vi "Add NI-XNET CAN Hardware_Create Disable Signal.vi"(7 "SysDef Ref":T1, 8 "error in (no error)":errorcluster, 10 "Disable Node Path":string, 11 "Signal Based Frame":refnum<k24>) -> (0 "error out":errorcluster, 3 "Signal Based Frame out":refnum<k24>)   [LabVIEW 2019, in "Simple SysDef API.lvlib"]
uses:
  <userlib>/SimpleSysDef/Simple SysDef API.lvlib
  <userlib>/SimpleSysDef/_SubVIs/System Definition Reference.ctl
  NationalInstruments.VeriStand.SystemDefinitionAPI
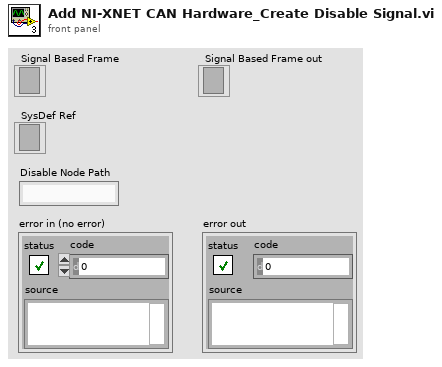
[diagram p1: front panel]
types:
  T1 = typedef "Simple SysDef API.lvlib/System Definition Reference.ctl" = refnum<k24>
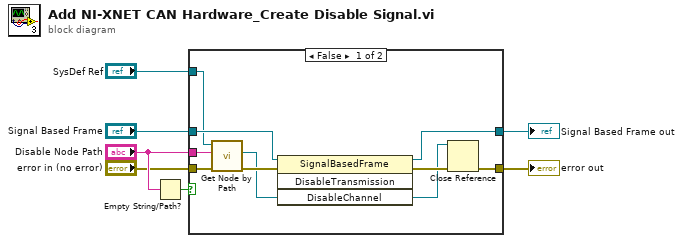
[diagram p0: block diagram]
diagram:
  n1 = Empty String/Path?(string/path="Disable Node Path") -> (empty?=w4:bool)
  n2 = case shown="False" w4 {
    tunnel: [w9 w18] -> w5
    tunnel: "Signal Based Frame" -> [w16 w17]
    tunnel: "error in (no error)" -> [w15 w18]
    tunnel: "Disable Node Path" -> [w14 _]
    tunnel: "SysDef Ref" -> [w12 _]
    tunnel: [w11 w17] -> w6
    frame False {
      n3 = call <userlib>:"Get Node by Path.vi"("error in (no error)"=w15, "System Definition Node Path"=w14, "SysDef Ref"=w12) -> ("error out"=w13:errorcluster, "Node Ref"=w8:refnum<k24>)  [unwired: 6 in, 1 out]
      n4 = invoke class="SignalBasedFrame" method="DisableTransmission"(reference=w16, error in=w13, "DisableChannel"=w8) -> (reference out=w11:refnum<k24>, error out=w10:errorcluster)  [unwired: 1 in, 2 out]
      n5 = Close Reference(reference=w8, error in (no error)=w10) -> (error out=w9:errorcluster)
    }
    frame True {
    }
  }
  "Signal Based Frame out" <- w6
  "error out" <- w5
